vi "Explorer_SplitPlotData.vi"(11 "Value":string) -> (1 "Data type":T1(ring), 3 "Array":dbl[](array[numeric]))   [LabVIEW 2022 SP3]
uses:
  <vilib>/Utility/error.llb/Trim Whitespace One-Sided.vi
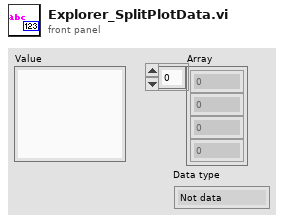
[diagram p1: front panel]
types:
  T1 = enum16{"Not data", "single values", "XY pairs", "Arrays"}
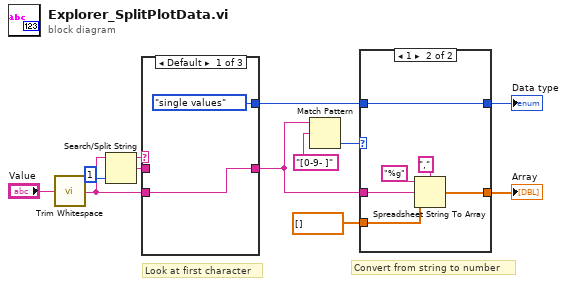
[diagram p0: block diagram]
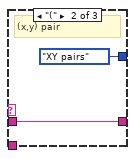
[diagram p2: hidden frame]
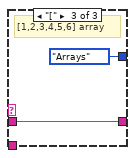
[diagram p3: hidden frame]
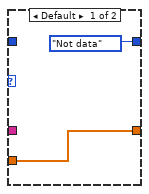
[diagram p4: hidden frame]
diagram:
  # "Convert from string to number"
  # "Look at first character"
  n1 = call <vilib>:"Trim Whitespace.vi"("string"="Value") -> ("trimmed string"=w3:string)  [unwired: 1 in]
  n2 = Search/Split String(string=w3, offset (0)=1) -> (substring before match=w6:string, match + rest of string=w5:string)  [unwired: 1 in, 1 out]
  n3 = case shown="Default" w6 {
    tunnel: w5 -> [_ w16 w18]
    tunnel: [w14 w16 w18] -> w4
    tunnel: w3 -> [w14 _ _]
    tunnel: [T1."single values" ("Data type") T1."XY pairs" ("Data type") T1."Arrays" ("Data type")] -> w2
    frame Default {
    }
    frame "(" {
      # "(x,y) pair"
    }
    frame "[" {
      # "[1,2,3,4,5,6] array"
    }
  }
  n4 = Match Pattern(string=w4, regular expression="[0-9- ]") -> (offset past match=w8:i32)  [unwired: 1 in, 3 out]
  n5 = case shown="1" w8 {
    tunnel: dbl[] [] -> [w20 w25]
    tunnel: [w20 w24] -> w11
    tunnel: w4 -> [_ w22]
    tunnel: [T1."Not data" ("Data type") w21] -> w1
    tunnel: w2 -> [_ w21]
    frame Default {
    }
    frame 1 {
      n6 = Spreadsheet String To Array(delimiter (Tab)=",", format string="%g", spreadsheet string=w22, array type (2D Dbl)=w25) -> (array=w24:dbl[])
    }
  }
  "Array" <- w11
  "Data type" <- w1
